vi "String to ExtendedComplex (Scalar).vi"(10 "Value (String)":string) -> (1 "Rest of string":string, 2 "Value (CXT)":cxt format="%#_13g", 3 "offset past number":i32)   [LabVIEW 2013, in "OpenScalar.lvlib"]
uses:
  OpenScalar.lvlib
  Get Decimal Separator.vi
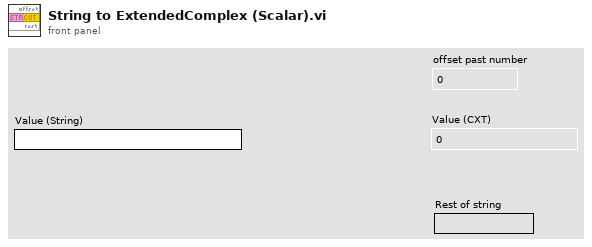
[diagram p1: front panel]
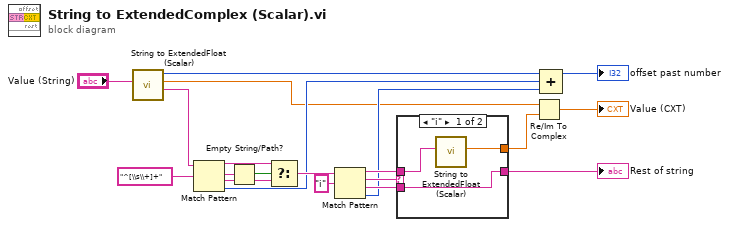
[diagram p0: block diagram]
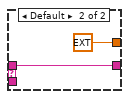
[diagram p2: hidden frame]
diagram:
  n1 = call "String to ExtendedFloat (Scalar).vi"("Value (String)"="Value (String)") -> ("Rest of string"=w2:string, "Value (Extended)"=w1:ext, "offset past number"=w3:i32)  [unwired: 8 in]
  n2 = Match Pattern(string=w2, regular expression="^[\\s\\+]+") -> (before substring=w9:string, match substring=w11:string, after substring=w8:string, offset past match=w5:i32)  [unwired: 1 in]
  n3 = Empty String/Path?(string/path=w11) -> (empty?=w10:bool)
  n4 = Select(t=w9, s=w10, f=w8) -> (s? t:f=w7:string)
  n5 = Match Pattern(string=w7, regular expression="i") -> (before substring=w16:string, match substring=w18:string, after substring=w14:string, offset past match=w6:i32)  [unwired: 1 in]
  n6 = case shown="\"i\"" w18 {
    tunnel: [w22 ext 0.0 ("y")] -> w17
    tunnel: w16 -> [w21 w24]
    tunnel: [w23 w24] -> w15
    tunnel: w14 -> [w23 _]
    frame "i" {
      n7 = call "String to ExtendedFloat (Scalar).vi"("Value (String)"=w21) -> ("Value (Extended)"=w22:ext)  [unwired: 8 in, 2 out]
    }
    frame Default {
    }
  }
  "Rest of string" <- w15
  n8 = Re/Im To Complex(1:w17, 2:w1) -> (0:→"Value (CXT)":cxt)
  n9 = Compound Arithmetic op=ADD(w3, w5, w6) -> (→"offset past number":i32)
